vi "Dashboard Main.vi"() -> ()   [LabVIEW 2015]
uses:
  <vilib>/Utility/miscctls.llb/LVRowAndColumnTypeDef.ctl
  <vilib>/event_ctls.llb/eventvkey.ctl
  <vilib>/Rock Robotics/Network Tables/NT Read Boolean.vi
  <vilib>/Rock Robotics/WPI/Dashboard/WPI_DashboardLogging Global.vi
  <vilib>/Utility/config.llb/Write Key (String).vi
  <vilib>/Utility/config.llb/Write Key (I32).vi
  <vilib>/Utility/config.llb/NI_LVConfig.lvlib
panel:
  out "Camera Image":T1(plugin-control)
  in  "Background":bool
  in  "TCP":refnum<k5>
  in  "Vision":u16(ring) items=["Camera Off", "USB Camera SW", "USB Camera HW", "IP Camera"]
  out "Camera IP":string
  out "Image Message":string="Timeout in Camera Communications"
  in  "Dashboard Tab":T2(tab)
  in  "AUTO Start Delay":dbl
  in  "AUTO Modes":T3(radio)
  in  "Select Auto":string(combo)
  out "NT Connection":bool
  in  "Camera Settings":T4={"Frame Rate"=30, "Compression"=30, "Size"=1} {"Frame Rate" scale=1.0..30.0; "Size" items=["640x480", "320x240", "160x120"]}
  out "Mode":T5(ring)=enum."Auto Disabled"
  in  "DB Camera Config":bool
  out "fps":dbl format="%#.1g"
  out "Mbps":dbl format="%#.1g"
  out "Mbps LED":bool
  in  "Rec Mode":enum32{"Stop", "Record", "Playback"}(radio)
  in  "DB/String 9":string
  in  "DB/String 8":string
  in  "DB/String 7":string
  in  "DB/String 6":string
  in  "DB/String 5":string
  in  "DB/String 4":string
  in  "DB/String 3":string
  in  "DB/String 2":string
  in  "DB/String 1":string
  in  "DB/String 0":string
  in  "DB/Slider 0":dbl(slide) scale=0.0..5.0
  in  "DB/Slider 1":dbl(slide) scale=0.0..5.0
  in  "DB/Slider 2":dbl(slide) scale=0.0..5.0
  in  "DB/Slider 3":dbl(slide) scale=0.0..5.0
  out "DB/LED 3":bool
  out "DB/LED 2":bool
  out "DB/LED 1":bool
  out "DB/LED 0":bool
  in  "DB/Button 3":bool
  in  "DB/Button 2":bool
  in  "DB/Button 1":bool
  in  "DB/Button 0":bool caption="New Name"
  out "Shooter Velocity":dbl
  in  "Shoot Duration":dbl=1000.0
  in  "Shoot speed":dbl=0.3
  out "Refreshed":bool
  in  "Refresh":bool
  out "Saved Level 3":dbl
  out "Saved Level 2":dbl
  out "Saved Level 1":dbl
  in  "Left Shooter RPM":dbl=5000.0
  out "Pot":dbl
  in  "Test Slider":dbl(slide) scale=0.0..100.0 scale format="%#_3g"
  in  "On/Off":bool caption="Solenoid"
  in  "Test Name":u16(ring) items=["Select the test to run..."]
  in  "Test Tree":string(tree)
  in  "Motor":cluster{"Value":dbl, "Enable":bool} {"Value" scale=-1.0..1.0 scale format="%#_3g"}
  out "Progress":T6 {"Test Progress" scale=0.0..100.0}
  in  "Rev/Fwd":cluster{"Forward":bool, "Reverse":bool}
  in  "Test Ring":u16(ring) items=["Monochrome", "Color"]
  out "Cmd Status":string
  in  "Execute Command":bool
  in  "Command Params":string[][](table)
  in  "Command Selection":i32(listbox)
  in  "CheckList":i32(listbox)
  out "Tree":string(tree)
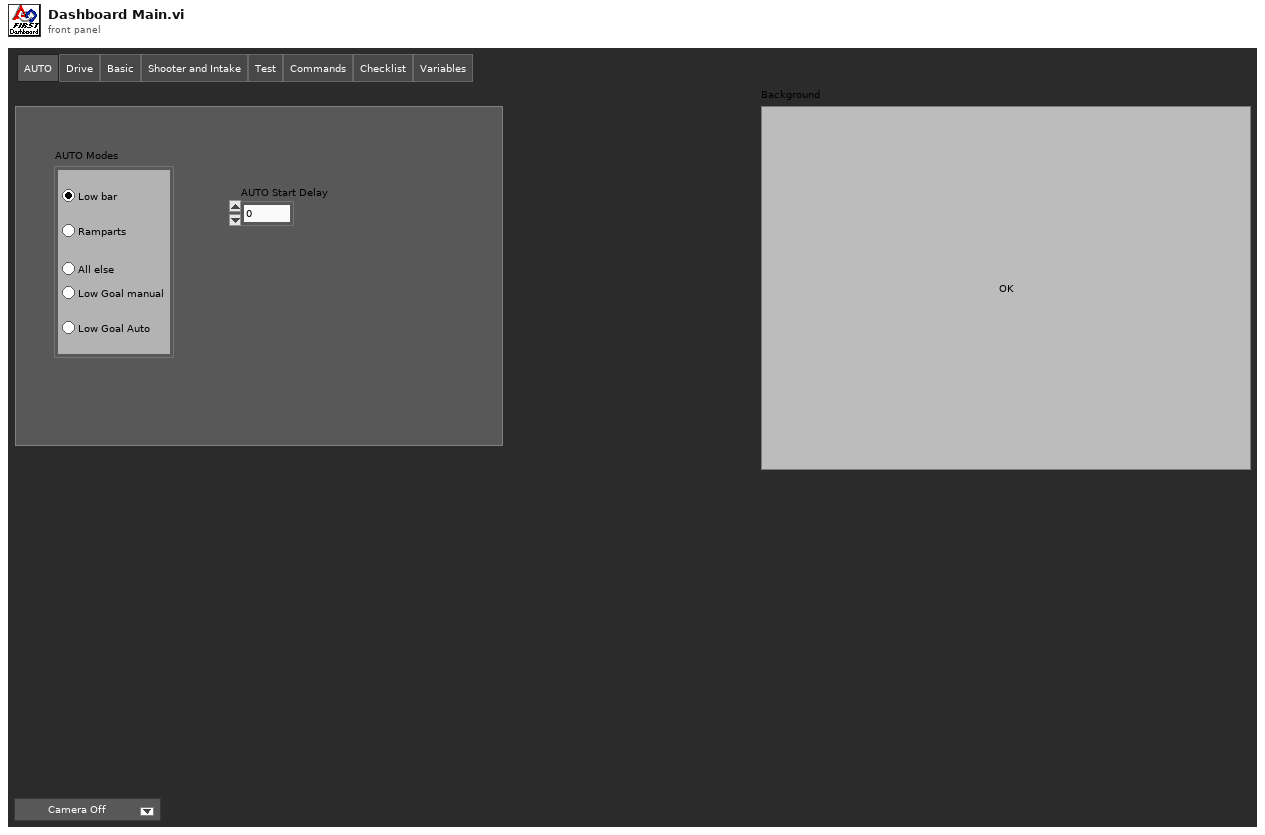
[diagram p1: front panel]
types:
  T1 = typedef "IMAQ Image.ctl" = refnum<image>
  T2 = enum32{"AUTO", "Drive", "Basic", "Shooter and Intake", "Test", "Commands", "Checklist", "Variables"}
  T3 = enum32{"Low bar", "Ramparts", "All else", "All else 2", "All else 3"}
  T4 = cluster{"Frame Rate":i32, "Compression":i32, "Size":u16}
  T5 = enum8{"Tele-Op Disabled", "Tele-Op Enabled", "Auto Disabled", "Auto Enabled", "Test Disabled", "Test Enabled", "Disconnected", "No Code", "E-Stop"}
  T6 = cluster{"Test Progress":u8, "Test Progress Text":string}
  T7 = cluster{"IDs":cluster{"RPC field ID":u16, "Unique ID":u16}, "String":string}
  T8 = enum32{"Drive", "Basic", "Custom", "Test", "Checklist", "Variables"}
  T9 = typedef "Image Type" = u32
  T10 = enum16{"open", "replace", "create", "open or create", "replace or create", "replace or create with confirmation"}
  T11 = cluster{"Camera Image":refnum<vi>, "Dashboard Tab":refnum<vi>, "Background":refnum<vi>, "Vision":refnum<vi>, "Rec Mode":refnum<vi>, "Test Slider":refnum<vi>, "On/Off ":refnum<vi>, "Test Ring":refnum<vi>, "Rev/Fwd":refnum<vi>, "Test Name":refnum<vi>, "Motor":refnum<vi>, "Progress":refnum<vi>, "CheckList":refnum<vi>, "Tree":refnum<vi>, "Test Tree":refnum<vi>, "Command Params":refnum<vi>, "Command Selection":refnum<vi>, "Execute Command":refnum<vi>, "Cmd Status":refnum<vi>}
  T12 = typedef "NI_LVConfig.lvlib/Config Data RefNum.ctl" = refnum<k1>
  T13 = cluster{"Error Strings":string, "Disable Counts":cluster{u16, u16}, "Rail Faults":cluster{u16, u16, u16}, "Robot IP":string, "DB Mode":u8, "Event Info":cluster{"Name":string, "Type":u8, "Number":u16, "Replay":u8}, "Camera Addr":string}
  T14 = cluster{"Storage":cluster{"Disk Free":u64, "RAM Block":u32, "RAM free":u32}, "CPU Utilization":cluster{"CPU % ISR":sgl, "CPU % Time Crit":sgl, "CPU % Timed Str":sgl, "CPU % High":sgl, "CPU % Above":sgl, "CPU % Normal":sgl, "CPU % Low":sgl}, "CAN":cluster{"% Bus Utilization":sgl, "Bus Off Cnt":u32, "TX_FIFO Full Cnt":u32, "Receive Error Cnt":u8, "Transmit Error Cnt":u8}, "HID":cluster{"HID Outputs":u32, "Rumble Low":u16, "Rumble High":u16}[]}
  T15 = cluster{"Status bits":cluster{"Test Mode":bool, "Autonomous":bool, "Enabled":bool, "Code Start":bool, "Brownout":bool, "Reserved 2":bool, "Reserved 3":bool, "E-Stop":bool}, "Code Trace":cluster{"Disabled":bool, "TeleOp":bool, "Auto":bool, "Test":bool}, "Controller Type":enum16{"unknown", "cRIO", "roboRio"}, "Code?":enum16{"unknown", "noCode", "code"}, "Battery V":dbl}
  T16 = cluster{"Control Bits":cluster{"TestMode":bool, "Autonomous":bool, "Enabled":bool, "FMS Present":bool, bool, bool, bool, "E-Stop":bool}, "Team Station ":u8, "Countdown":sgl, "Joystick Values":cluster{"Axes":dbl[], "Buttons":bool[], "POVs":i16[]}[]}
  T17 = cluster{"Operation":enum16{"Update", "Clear"}, "Color Box":u32}[]
  T18 = typedef "eventvkey.ctl" = enum16{"ASCII", "Enter", "Return", "Shift", "Ctrl", "Alt", "Cmd", "Opt", "Caps", "NumLock", "Clear", "Break", "Up", "Down", "Left", "Right", "Insert", "Delete", "Home", "End", "PageUp", "PageDown", "Escape", "Help", "Pause", "ScrollLock", "F1", "F2", "F3", "F4", "F5", "F6", "F7", "F8", "F9", "F10", "F11", "F12", "F13", "F14", "F15", "F16", "F17", "F18", "F19", "F20", "F21", "F22", "F23", "F24", "Play", "VolumeUp", "VolumeDown", "Mute", "Two Byte Char"}
  T19 = cluster{"Image Size":bool, "Image Type":bool, "Pixel Value":bool, "ROI Information":bool, "Zoom Factor":bool}
  T20 = enum8{"Enabled", "Disabled", "Disabled and Grayed Out"}
  T21 = cluster{"Operation":enum16{"Update", "Clear"}, "Color Box":u32}
  T22 = typedef "LVRowAndColumnTypeDef.ctl" = cluster{"Row":i32, "Column":i32}
  T23 = cluster{"Shift":bool, "Ctrl":bool, "Alt":bool, "Cmd":bool, "Opt":bool}
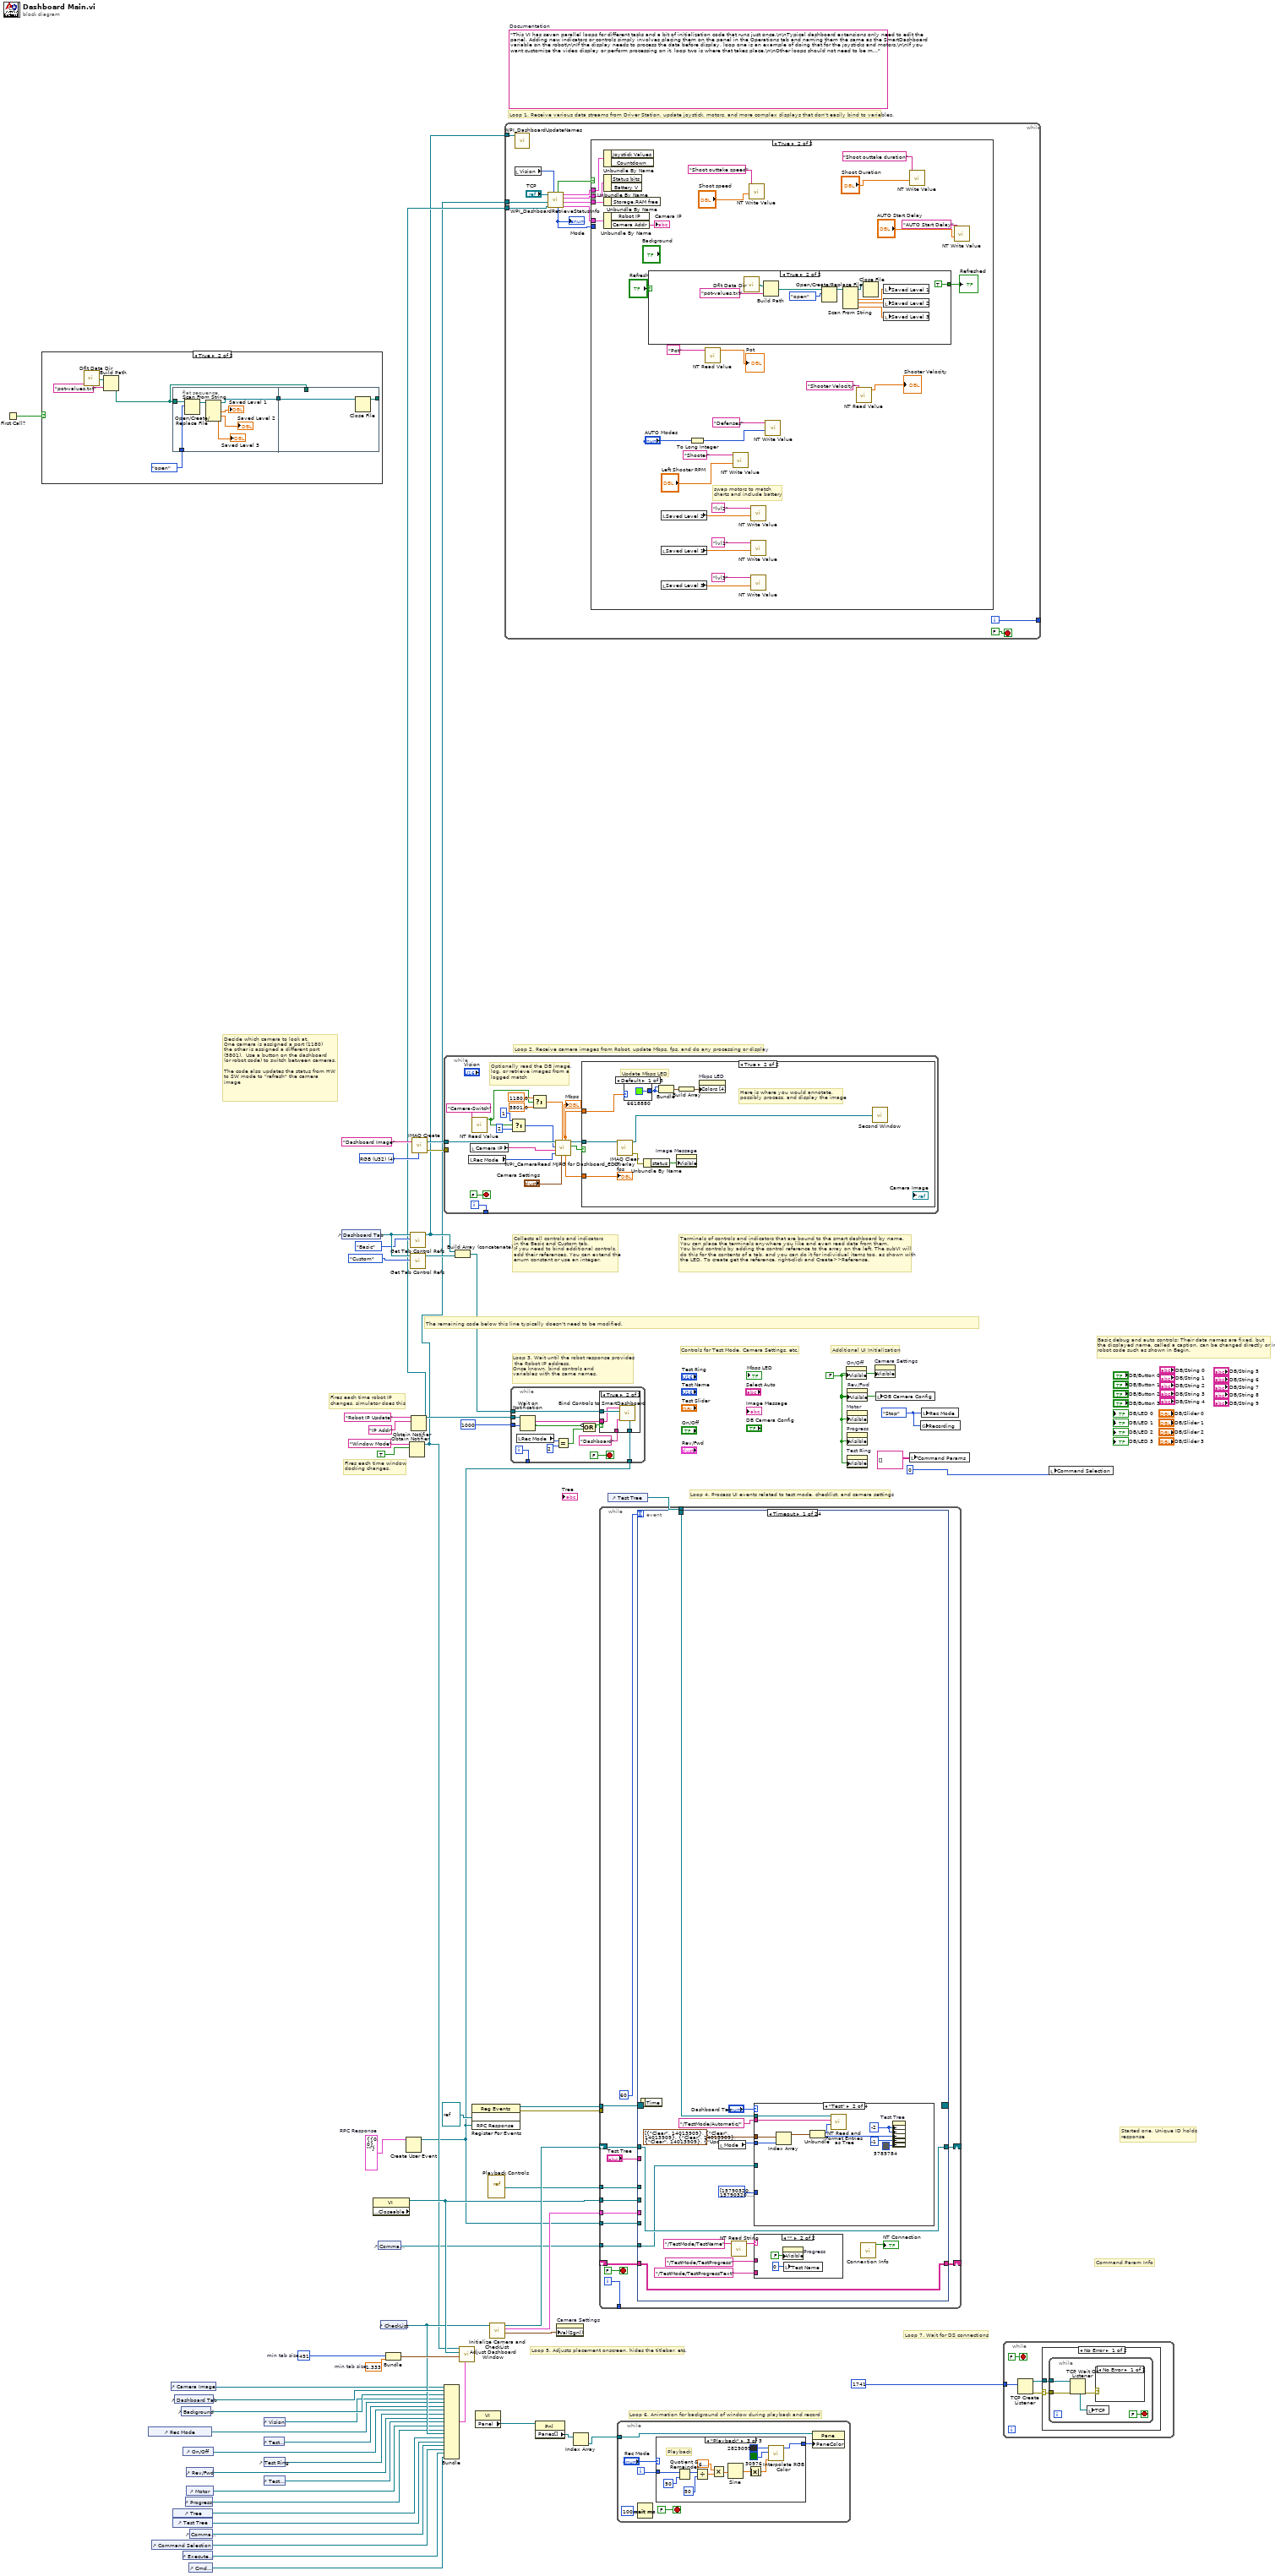
[diagram p0: block diagram]
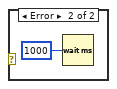
[diagram p3: hidden frame]
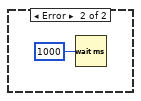
[diagram p4: hidden frame]
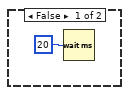
[diagram p5: hidden frame]
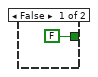
[diagram p6: hidden frame]
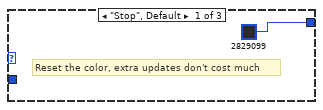
[diagram p7: hidden frame]
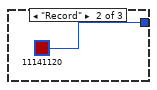
[diagram p8: hidden frame]
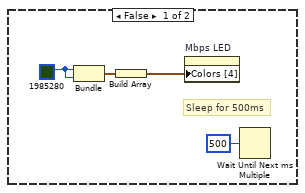
[diagram p10: hidden frame]
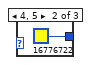
[diagram p11: hidden frame]
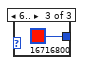
[diagram p12: hidden frame]
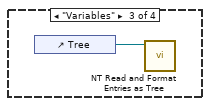
[diagram p14: hidden frame]
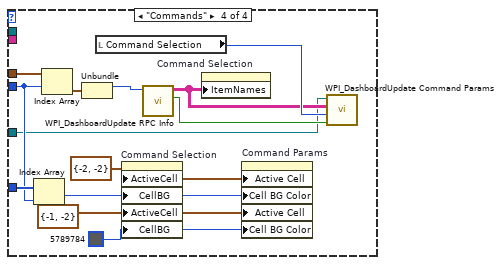
[diagram p15: hidden frame]
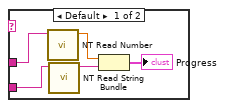
[diagram p16: hidden frame]
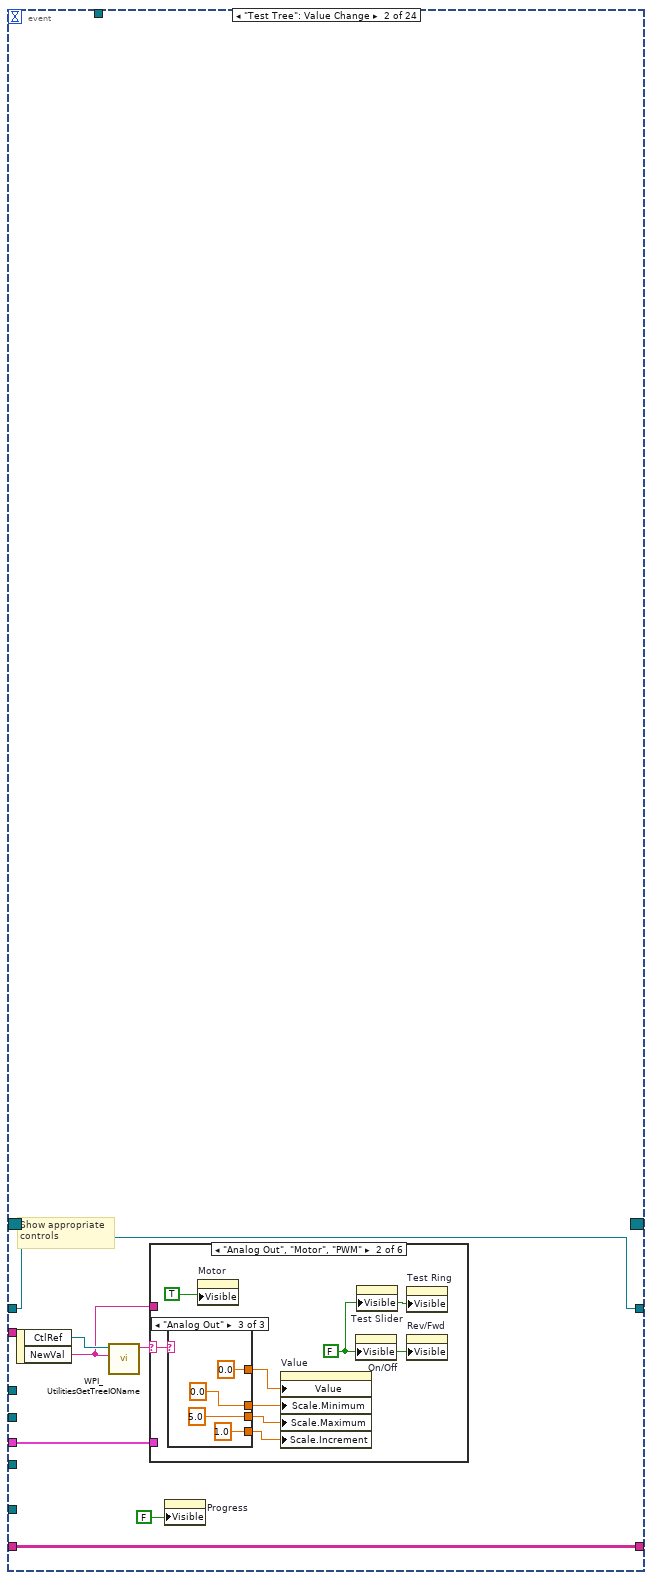
[diagram p17: hidden frame]
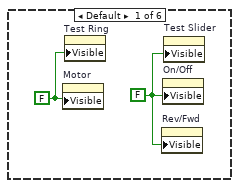
[diagram p18: hidden frame]
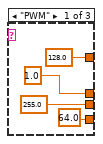
[diagram p19: hidden frame]
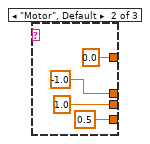
[diagram p20: hidden frame]
diagram:
  w12 = T7 {"IDs"={"RPC field ID"=0, "Unique ID"=0}, "String"=""}  # RPC Response
  w35 = 491  # min tab size
  w34 = 1.333  # min tab size
  w41 = enum32{"Stop", "Record", "Playback"}."Stop" ("Rec Mode")
  w19 = FALSE ("Visible")
  (unwired) "This VI has seven parallel loops for different tasks and a bit of initialization code that runs just once.\n\nTypical dashboard extensions only need to edit the panel. Adding new indicators or controls simply involves placing them on the panel in the Operations tab and naming them the same as the SmartDashboard variable on the robot\n\nIf the display needs to process the data before display, loop one is an example of doing that for the joysticks and motors.\n\nIf you want customize the video display or perform processing on it, loop two is where that takes place.\n\nOther loops should not need to be modified. They are pretty standard, and document the task they perform."  # Documentation
  w61 = T9 4 items=["Grayscale (U8)", "Grayscale (I16)", "Grayscale (SGL)", "Complex (CSG)", "RGB (U32)", "HSL (U32)", "RGB (U64)"] ("Image Type")
  # "Decide which camera to look at.\nOne camera is assigned a port (1180)\nthe other is assigned a different port\n(5801).  Use a button on the dashboard\n(or robot code) to switch between cameras.\n\nThe code also updates the status from HW\nto SW mode to \"refresh\" the camera\nimage"
  # "Command Param Info"
  # "Started one, Unique ID holds\nresponse"
  # "Loop 7. Wait for DS connections"
  # "Basic debug and auto controls: Their data names are fixed, but\nthe displayed name, called a caption, can be changed directly or in\nrobot code such as shown in Begin."
  # "Controls for Test Mode, Camera Settings, etc."
  # "Additional UI Initialization"
  # "Loop 6. Animation for background of window during playback and record"
  # "Fires each time robot IP\nchanges, simulator does this"
  # "Fires each time window\ndocking changes."
  # "Collects all controls and indicators\nin the Basic and Custom tab.\nIf you need to bind additional controls,\nadd their references. You can extend the\nenum constant or use an integer."
  # "The remaining code below this line typically doesn't need to be modified."
  # "Loop 4. Process UI events related to test mode, checklist, and camera settings"
  # "Terminals of controls and indicators that are bound to the smart dashboard by name.\nYou can place the terminals anywhere you like and even read data from them.\nYou bind controls by adding the control reference to the array on the left. The subVI will\ndo this for the contents of a tab, and you can do it for individual items too, as shown with\nthe LED. To create get the reference, right-click and Create>>Reference."
  # "Loop 3. Wait until the robot response provides\n the Robot IP address.\nOnce known, bind controls and\nvariables with the same names."
  # "Loop 5. Adjusts placement onscreen, hides the titlebar, etc."
  # "Loop 1. Receive various data streams from Driver Station, update joystick, motors, and more complex displays that don't easily bind to variables."
  # "Loop 2. Receive camera images from Robot, update Mbps, fps, and do any processing or display"
  n1 = First Call?() -> (First Call?: T/F=w1:bool)
  n2 = case shown="True" w1 {
    frame False {
    }
    frame True {
      n3 = call <vilib>:"Dflt Data Dir.vi"() -> ("App:Default Data Directory"=w66:path)
      n4 = Build Path(base path=w66, name or relative path="pot-values.txt") -> (appended path=w63:path)
      n5 = flat-sequence {
        tunnel: w63 -> [w73]
        tunnel: T10."open" ("operation (0:open)") -> [w72]
        tunnel: [w67] -> w62
        tunnel: [w75] -> _
        tunnel: w63 -> [_]
        tunnel: w62 -> [w74]
        frame #0 {
          n6 = Open/Create/Replace File(file path (use dialog)=w73, operation (0:open)=w72) -> (refnum out=w71:refnum<file>)  [unwired: 4 in, 2 out]
          n7 = Scan From String(w71) -> (w67:refnum<file>, output 1=→"Saved Level 1":dbl, output 2=→"Saved Level 2":dbl, output 3=→"Saved Level 3":dbl)  [unwired: 5 in, 1 out]
        }
        frame #1 {
          n8 = Close File(refnum=w74) -> (path=w75:path)  [unwired: 1 in, 1 out]
        }
      }
    }
  }
  n9 = control-ref of="Rec Mode"() -> (w25:refnum<vi>)
  n10 = control-ref of="Command Selection"() -> (w11:refnum<vi>)
  n11 = control-ref of="Camera Image"() -> (w3:refnum<vi>)
  n12 = control-ref of="Tree"() -> (w29:refnum<vi>)
  n13 = control-ref of="Test Tree"() -> (w28:refnum<vi>)
  n14 = control-ref of="Dashboard Tab"() -> (w36:refnum<vi>)
  n15 = control-ref of="Background"() -> (w5:refnum<vi>)
  n16 = control-ref of="Execute Command"() -> (w13:refnum<vi>)
  n17 = control-ref of="On/Off"() -> (w23:refnum<vi>)
  n18 = control-ref of="Progress"() -> (w20:refnum<vi>)
  n19 = control-ref of="Rev/Fwd"() -> (w21:refnum<vi>)
  n20 = control-ref of="Motor"() -> (w26:refnum<vi>)
  n21 = control-ref of="Cmd Status"() -> (w7:refnum<vi>)
  n22 = control-ref of="Command Params"() -> (w14:refnum<vi>)
  n23 = control-ref of="Test Slider"() -> (w24:refnum<vi>)
  n24 = control-ref of="Vision"() -> (w4:refnum<vi>)
  n25 = control-ref of="Test Ring"() -> (w22:refnum<vi>)
  n26 = control-ref of="Test Name"() -> (w27:refnum<vi>)
  n27 = control-ref of="Dashboard Tab"() -> (w39:refnum<vi>)
  n28 = property class="VI" props=["Front Panel.Closeable"]() -> (reference out=w40:refnum<vi>)  [unwired: 2 in, 2 out]
  n29 = control-ref of="Command Params"() -> (w6:refnum<vi>)
  n30 = control-ref of="CheckList"() -> (w30:refnum<vi>)
  n31 = Bundle("min tab size"=w35, "min tab size"=w34) -> (w33:cluster{"min tab size":i32, "min tab size":dbl})  [unwired: 1 in]
  n32 = Create User Event(user event datatype=w12) -> (user event=w8:refnum<user-event>)  [unwired: 1 in, 1 out]
  n33 = Obtain Notifier(name (unnamed)="Window Mode", notification data type=TRUE) -> (notifier out=w16:refnum<notifier>)  [unwired: 2 in, 2 out]
  n34 = call <vilib>:"Get Tab Control Refs.vi"("Page Index"=T8."Basic" ("Dashboard Tab"), "TabControl in"=w39) -> ("ControlsOnPage"=w17:refnum<vi>[])  [unwired: 9 in]
  n35 = call <vilib>:"Get Tab Control Refs.vi"("Page Index"=T8."Custom" ("Dashboard Tab"), "TabControl in"=w39) -> ("ControlsOnPage"=w38:refnum<vi>[])  [unwired: 9 in]
  n36 = Obtain Notifier(name (unnamed)="Robot IP Update", notification data type="IP Addr" ("name (unnamed)")) -> (notifier out=w18:refnum<notifier>)  [unwired: 2 in, 2 out]
  n37 = call "IMAQ Create"("Image Name"="Dashboard Image", "Image Type"=w61) -> ("New Image"=w59:T1, "error out"=w58:errorcluster)  [unwired: 2 in, 1 out]
  n38 = while {
    tunnel: w59 -> [w91]
    tunnel: w58 -> [_]
    tunnel: [w92] -> _
    i -> [w92]
    stop <- FALSE stop-if-true
    # "Optionally read the DB image,\nlog, or retrieve images from a\nlogged match"
    n39 = local read "Rec Mode"() -> (w86:enum32{"Stop", "Record", "Playback"})
    n40 = local read "Camera IP"() -> (w85:string)
    n41 = call-poly <vilib>:"NT Read Value.vi"("Name"="Camera-Switch") -> ("Boolean"=w76:bool)  [unwired: 9 in, 1 out]
    n42 = Select(t=1, s=w76, f=2) -> (s? t:f=w81:i32)
    n43 = Select(t=1180.0, s=w76, f=5801.0) -> (s? t:f=w80:dbl)
    n44 = call "WPI_CameraRead MJPG for Dashboard_EDIT.vi"("Camera Settings"="Camera Settings", "Camera Port"=w80, "Rec Mode"=w86, "Camera IP"=w85, "Camera Mode"=w81, "Refnum in"=w91) -> ("Active"=w89:bool, "Refnum out"=w90:T1, "FPS"=w88:dbl, "Bandwidth (Mbps)"=w84:dbl)  [unwired: 2 in]
    "Mbps" <- w84
    n45 = case shown="True" w89 {
      tunnel: w90 -> [_ w101]
      tunnel: w84 -> [_ w100]
      tunnel: w88 -> [_ w99]
      frame False {
        w94 = u32 1985280 ("Color Box")
        # "Sleep for 500ms"
        n46 = Bundle("Color Box"=w94, "Color Box"=w94) -> (w96:cluster{"Color Box":u32, "Color Box":u32})  [unwired: 1 out]
        n47 = Build Array(w96) -> (w95:cluster{"Color Box":u32, "Color Box":u32}[])
        n48 = property on="Mbps LED" class="Bool (strict)"("Colors [4]"=w95) -> ()  [unwired: 2 in, 2 out]
        n49 = Wait Until Next ms Multiple(millisecond multiple=u32 500) -> ()  [unwired: 1 out]
      }
      frame True {
        # "Here is where you would annotate,\npossibly process, and display the image"
        # "Update Mbps LED"
        n50 = call "IMAQ Clear Overlay"("Image"=w101) -> ("error out"=w105:errorcluster, "Image Out"=w98:T1)  [unwired: 2 in, 7 out]
        n51 = case shown="Default" w100 {
          tunnel: [u32 6618880 ("Color Box") u32 16776722 ("Color Box") u32 16716800 ("Color Box")] -> w102
          frame Default {
          }
          frame 4, 5 {
          }
          frame 6.. {
          }
        }
        n52 = Unbundle By Name(w105) -> ("status"=w106:bool)
        n53 = Bundle("Color Box"=w102, "Color Box"=w102) -> (w104:cluster{"Color Box":u32, "Color Box":u32})  [unwired: 1 out]
        n54 = property on="Image Message" class="Str"("Visible"=w106) -> ()  [unwired: 2 in, 2 out]
        n55 = Build Array(w104) -> (w103:cluster{"Color Box":u32, "Color Box":u32}[])
        n56 = property on="Mbps LED" class="Bool (strict)"("Colors [4]"=w103) -> ()  [unwired: 2 in, 2 out]
        n57 = call "Second Window.vi"("Input Camera Image"=w98) -> ()  [unwired: 1 in]
        "fps" <- w99
      }
    }
  }
  n58 = Bundle("Camera Image"=w3, "Dashboard Tab"=w36, "Background"=w5, "Vision"=w4, "Rec Mode"=w25, "Test Slider"=w24, "On/Off"=w23, "Test Ring"=w22, "Rev/Fwd"=w21, "Test Name"=w27, "Motor"=w26, "Progress"=w20, "CheckList"=w30, "Tree"=w29, "Test Tree"=w28, "Command Params"=w14, "Command Selection"=w11, "Execute Command"=w13, "Cmd Status"=w7) -> (w2:T11)  [unwired: 1 in]
  n59 = Build Array (concatenate)(w17, w38) -> (w37:refnum<vi>[])
  n60 = call "Adjust Dashboard Window.vi"("Sizing Refnums"=w2, "Size Constraints"=w33, "VI"=w40, "WIn Mode"=w16) -> ()  [unwired: 8 in]
  n61 = register-events(refnum<vi> refnum, w8) -> (reference out=w45:refnum<event-registration>, error out=w44:errorcluster)  [unwired: 2 in]
  n62 = property class="VI"() -> ("Panel"=w48:refnum<vi>)  [unwired: 2 in, 2 out]
  n63 = vi-ref "Playback Controls.vi"() -> (w46:refnum<vi>)
  n64 = call "Initialize Camera and CheckList.vi"("ListBox in"=w30) -> ("Cluster"=w52:cluster{"value":i32, "value":i32, "index":i32}, "Array"=w53:cluster{string[]}[], "File Refnum"=w51:T12)  [unwired: 8 in]
  n65 = while {
    tunnel: [w121] -> _
    tunnel: w18 -> [w115]
    tunnel: w17 -> [w114]
    tunnel: w16 -> [w110]
    i -> [w121]
    stop <- FALSE stop-if-true
    n66 = call <vilib>:"WPI_DashboardUpdateNames.vi"("Controls on Tab"=w114) -> ()  [unwired: 11 in]
    n67 = local read "Vision"() -> (w112:u16)
    n68 = call <vilib>:"WPI_DashboardRetrieveStatusInfo.vi"("Vision"=w112, "Binding Refnum"=w115, "Window Mode Notifier"=w110, "TCP Cnx"="TCP") -> ("Power and Errors"=w116:T13, "Robot Metrics"=w119:T14, "Status Info"=w120:T15, "Control Info"=w117:T16, "Robot Mode"=w113:T5, "Process?"=w118:bool)  [unwired: 2 in]
    "Mode" <- w113
    n69 = case shown="True" w118 {
      tunnel: w120 -> [_ w151]
      tunnel: w119 -> [_ w150]
      tunnel: w117 -> [_ w149]
      tunnel: w116 -> [_ w148]
      tunnel: w113 -> [_ _]
      frame False {
        n70 = Wait (ms)(milliseconds to wait=u32 20) -> ()  [unwired: 1 out]
      }
      frame True {
        # "swap motors to match\ncharts and include battery"
        n71 = Unbundle By Name(w149) -> ()  [unwired: 2 out]
        n72 = Unbundle By Name(w151) -> ()  [unwired: 2 out]
        n73 = Unbundle By Name(w150) -> ()  [unwired: 1 out]
        n74 = Unbundle By Name(w148) -> ("Camera Addr"=→"Camera IP":string)  [unwired: 1 out]
        n75 = case shown="True" "Refresh" {
          tunnel: [FALSE TRUE] -> w133
          frame False {
          }
          frame True {
            n76 = call <vilib>:"Dflt Data Dir.vi"() -> ("App:Default Data Directory"=w161:path)
            n77 = Build Path(base path=w161, name or relative path="pot-values.txt") -> (appended path=w159:path)
            n78 = Open/Create/Replace File(file path (use dialog)=w159, operation (0:open)=T10."open") -> (refnum out=w162:refnum<file>)  [unwired: 4 in, 2 out]
            n79 = Scan From String(w162) -> (w154:refnum<file>, output 1=w155:dbl, output 2=w157:dbl, output 3=w156:dbl)  [unwired: 5 in, 1 out]
            n80 = Close File(refnum=w154) -> ()  [unwired: 1 in, 2 out]
            n81 = local write "Saved Level 1"(w155) -> ()
            n82 = local write "Saved Level 2"(w157) -> ()
            n83 = local write "Saved Level 3"(w156) -> ()
          }
        }
        "Refreshed" <- w133
        n84 = local read "Saved Level 2"() -> (w135:dbl)
        n85 = local read "Saved Level 1"() -> (w134:dbl)
        n86 = local read "Saved Level 3"() -> (w136:dbl)
        n87 = To Long Integer(number="AUTO Modes") -> (32bit integer=w138:i32)
        n88 = call-poly <vilib>:"NT Read Value.vi"("Name"="Pot") -> ("Numeric"=→"Pot":dbl)  [unwired: 9 in, 1 out]
        n89 = call-poly <vilib>:"NT Write Value.vi"("Numeric"="Left Shooter RPM", "Name"="Shooter") -> ()  [unwired: 9 in, 1 out]
        n90 = call-poly <vilib>:"NT Write Value.vi"("Numeric"="Shoot speed", "Name"="Shoot outtake speed") -> ()  [unwired: 9 in, 1 out]
        n91 = call-poly <vilib>:"NT Write Value.vi"("Numeric"=w135, "Name"="lvl2") -> ()  [unwired: 9 in, 1 out]
        n92 = call-poly <vilib>:"NT Write Value.vi"("Numeric"=w134, "Name"="lvl1") -> ()  [unwired: 9 in, 1 out]
        n93 = call-poly <vilib>:"NT Write Value.vi"("Numeric"=w136, "Name"="lvl3") -> ()  [unwired: 9 in, 1 out]
        n94 = call-poly <vilib>:"NT Write Value.vi"("Numeric"=w138, "Name"="Defenses") -> ()  [unwired: 9 in, 1 out]
        n95 = call-poly <vilib>:"NT Read Value.vi"("Name"="Shooter Velocity") -> ("Numeric"=→"Shooter Velocity":dbl)  [unwired: 9 in, 1 out]
        n96 = call-poly <vilib>:"NT Write Value.vi"("Numeric"="Shoot Duration", "Name"="Shoot outtake duration") -> ()  [unwired: 9 in, 1 out]
        n97 = call-poly <vilib>:"NT Write Value.vi"("Numeric"="AUTO Start Delay", "Name"="AUTO Start Delay") -> ()  [unwired: 9 in, 1 out]
      }
    }
  }
  n98 = while {
    tunnel: w37 -> [w175]
    tunnel: w18 -> [w173]
    tunnel: [w171] -> _
    tunnel: u32 1000 ("milliseconds to wait") -> [w170]
    tunnel: w8 -> [w163]
    i -> [w171]
    stop <- FALSE stop-if-true
    n99 = local read "Rec Mode"() -> (w166:enum32{"Stop", "Record", "Playback"})
    n100 = Wait on Notification(notifier=w173, timeout in ms (-1)=w170) -> (notification=w172:string, timed out?=w168:bool)  [unwired: 2 in, 2 out]
    n101 = Equal?(x=w166, y=u16 2 ("Rec Mode")) -> (x = y?=w167:bool)
    n102 = Compound Arithmetic op=OR(invert w168, w167) -> (w169:bool)
    n103 = case shown="True" w169 {
      tunnel: w175 -> [_ w179]
      tunnel: w172 -> [_ w178]
      tunnel: "Dashboard" -> [_ w177]
      tunnel: w163 -> [_ w176]
      frame False {
      }
      frame True {
        n104 = call <vilib>:"Bind Controls to SmartDashboard.vi"("RPC ref"=w176, "Client Name"=w177, "Bound Control Refs"=w179, "Server IP Address"=w178) -> ()  [unwired: 8 in]
      }
    }
  }
  n105 = property class="Pnl"(reference=w48) -> ("Panes[]"=w49:refnum<vi>[])  [unwired: 1 in, 2 out]
  n106 = property on="Camera Settings" class="Clust (strict)"("Val(Sgnl)"=w52) -> ()  [unwired: 2 in, 2 out]
  n107 = Index Array(array=w49) -> (element=w47:refnum<vi>)  [unwired: 1 in]
  n108 = control-ref of="Test Tree"() -> (w50:refnum<vi>)
  n109 = while {
    tunnel: w53 -> [w191]
    shift-right: [w190] -> _
    shift-left: w51 -> [w189]
    tunnel: [w188] -> _
    tunnel: w50 -> [w187]
    tunnel: w46 -> [w186]
    tunnel: w45 -> [w185]
    tunnel: w44 -> [_]
    tunnel: w40 -> [w184]
    tunnel: w8 -> [w183]
    tunnel: w6 -> [w182]
    shift-right: [w181] -> _
    shift-left: _ -> [w180]
    i -> [w188]
    stop <- FALSE stop-if-true
    n110 = event shown="[0] Timeout" {
      selector: w185 -> [_ _ _ _ _ _ _ _ _ _ _ _ _ _ _ _ _ _ _ _ _ _ _ _]
      dyn-events: [_ _ _ _ _ _ _ _ _ _ _ _ _ _ _ _ _ _ w498 _ _ _ _ _] -> _
      timeout: u32 60 ("milliseconds to wait") -> [_ _ _ _ _ _ _ _ _ _ _ _ _ _ _ _ _ _ _ _ _ _ _ _]
      tunnel: w187 -> [w204 _ _ _ _ _ _ _ _ _ _ _ _ _ _ _ _ _ _ _ _ _ _ _]
      tunnel: "Test Tree" -> [_ _ _ _ _ _ _ _ _ _ _ _ _ w463 w472 w475 w480 w489 _ _ _ _ _ _]
      tunnel: w191 -> [_ w242 _ _ _ _ _ _ _ _ _ w425 w456 _ _ _ _ _ _ _ _ _ _ _]
      tunnel: [w201 w241 w345 w351 w361 w365 w371 w383 w391 w397 w410 w424 w449 w462 w470 w474 w479 w488 w500 w516 w518 w526 w537 w542] -> w190
      tunnel: w189 -> [w201 w241 w345 w351 w361 w365 w371 w383 w391 w397 w410 w423 w449 w462 w470 w474 w479 w488 w500 w516 w518 w526 w537 w542]
      tunnel: w186 -> [_ _ _ _ _ _ _ _ _ _ _ _ _ _ _ _ _ _ w501 _ w521 _ _ _]
      tunnel: w184 -> [_ _ _ _ _ _ _ _ _ _ _ _ _ _ _ _ _ _ w496 _ _ _ _ _]
      tunnel: w183 -> [_ _ _ _ _ _ _ _ _ _ _ _ _ _ _ _ _ _ w494 _ _ _ _ _]
      tunnel: w182 -> [w196 _ _ _ _ _ w369 _ _ _ _ _ _ _ _ _ _ _ _ _ _ _ _ _]
      tunnel: [w195 w240 w344 w350 w360 w366 w367 w377 w388 w396 w409 w422 w448 w461 w469 w473 w478 w487 w493 w514 w517 w522 w530 w543] -> w181
      tunnel: w180 -> [w195 w240 w344 w350 w360 w366 w367 _ _ w396 w409 w422 w448 w461 w469 w473 w478 w487 w493 w514 w517 w522 w530 w543]
      event Timeout {
        n111 = event-data() -> ()  [unwired: 1 in, 1 out]
        n112 = local read "Mode"() -> (w198:T5)
        n113 = call <vilib>:"NT Read String.vi"("Name"="/TestMode/TestName") -> ("String"=w207:string)  [unwired: 9 in, 1 out]
        n114 = case shown="\"Test\"" "Dashboard Tab" {
          tunnel: w204 -> [_ w218 _ _]
          tunnel: "/TestMode/Automatic/" ("Name Pattern") -> [_ w217 _ _]
          tunnel: T17 [{"Operation"=enum."Clear", "Color Box"=14013909}, {"Operation"=enum."Clear", "Color Box"=14013909}, {"Operation"=enum."Clear", "Color Box"=14013909}, {"Operation"=enum."Clear", "Color Box"=14013909}, {"Operation"=enum."Update", "Color Box"=14013909}, {"Operation"=enum."Update", "Color Box"=16777215}, {"Operation"=enum."Clear", "Color Box"=14013909}, {"Operation"=enum."Clear", "Color Box"=14013909}, {"Operation"=enum."Clear", "Color Box"=14013909}] -> [_ w210 _ w227]
          tunnel: w198 -> [_ w209 _ w226]
          tunnel: u32[] [15790320, 15790320, 15790320, 15790320, 16777215, 16777215, 15790320, 15790320, 15790320] -> [_ _ _ w232]
          tunnel: w196 -> [_ _ _ w220]
          frame "Shooter and Intake", Default {
          }
          frame "Test" {
            w216 = -2 ("Active Item:Row Number")
            n115 = Index Array(array=w210, index=w209) -> (element=w211:T21)
            n116 = Unbundle(w211) -> ("Operation"=w212:enum16{"Update", "Clear"}, "Color Box"=w213:u32)
            n117 = call <vilib>:"NT Read and Format Entries as Tree.vi"("Operation"=w212, "Name Pattern"=w217, "Tree Refnum"=w218) -> ()  [unwired: 7 in, 2 out]
            n118 = property on="Test Tree" class="Tree (strict)"("Active Item Row Number"=w216, "ActiveColNum"=w216, "CellBG"=w213, "Active Item Row Number"=-1 ("Active Item:Row Number"), "CellBG"=u32 5789784 ("Color Box")) -> ()  [unwired: 2 in, 2 out]
          }
          frame "Variables" {
            n119 = control-ref of="Tree"() -> (w219:refnum<vi>)
            n120 = call <vilib>:"NT Read and Format Entries as Tree.vi"("Tree Refnum"=w219) -> ()  [unwired: 9 in, 2 out]
          }
          frame "Commands" {
            w228 = u32 5789784 ("Color Box")
            w229 = T22 {"Row"=-1, "Column"=-2} ("Active Cell:Active Cell")
            w231 = T22 {"Row"=-2, "Column"=-2} ("Active Cell:Active Cell")
            n121 = Index Array(array=w232, index=w226) -> (element=w230:u32)
            n122 = Index Array(array=w227, index=w226) -> (element=w225:T21)
            n123 = Unbundle(w225) -> ("Operation"=w224:enum16{"Update", "Clear"})  [unwired: 1 out]
            n124 = local read "Command Selection"() -> (w223:i32)
            n125 = property on="Command Selection" class="MCListbox (strict)"("ActiveCell"=w231, "CellBG"=w230, "ActiveCell"=w229, "CellBG"=w228) -> ()  [unwired: 2 in, 2 out]
            n126 = call <vilib>:"WPI_DashboardUpdate RPC Info.vi"("Operation"=w224) -> ("update"=w222:bool, "commands"=w221:string[][])  [unwired: 9 in]
            n127 = property on="Command Selection" class="MCListbox (strict)"("ItemNames"=w221) -> ()  [unwired: 2 in, 2 out]
            n128 = property on="Command Params" class="Tbl (strict)"("Active Cell"=w231, "Cell BG Color"=w230, "Active Cell"=w229, "Cell BG Color"=w228) -> ()  [unwired: 2 in, 2 out]
            n129 = call <vilib>:"WPI_DashboardUpdate Command Params.vi"("Update"=w222, "NewVal"=w223, "Commands"=w221, "Param Tbl"=w220) -> ()  [unwired: 7 in, 1 out]
          }
        }
        n130 = case shown="\"\"" w207 {
          tunnel: "/TestMode/TestProgress" ("Name") -> [w234 _]
          tunnel: "/TestMode/TestProgressText" ("Name") -> [w233 _]
          frame Default {
            n131 = call <vilib>:"NT Read Number.vi"("Name"=w234) -> ("Numeric"=w235:dbl)  [unwired: 9 in, 1 out]
            n132 = call <vilib>:"NT Read String.vi"("Name"=w233) -> ("String"=w236:string)  [unwired: 9 in, 1 out]
            n133 = Bundle("Numeric"=w235, "String"=w236) -> (→"Progress":cluster{"Numeric":dbl, "String":string})  [unwired: 1 in]
          }
          frame "" {
            n134 = property on="Progress" class="Clust (strict)"("Visible"=FALSE) -> ()  [unwired: 2 in, 2 out]
            n135 = local write "Test Name"(u16 0) -> ()
          }
        }
        n136 = call <vilib>:"Connextion Info.vi"() -> ("Connected"=→"NT Connection":bool)  [unwired: 10 in, 1 out]
      }
      event "Test Tree": Value Change {
        # "Show appropriate\ncontrols"
        n137 = event-data() -> ("CtlRef"=w245:refnum<vi>, "NewVal"=w243:string)  [unwired: 1 in]
        n138 = call <vilib>:"WPI_UtilitiesGetTreeIOName.vi"("NewVal"=w243, "TreeControl in"=w245) -> ("I/O Name"=w246:string)  [unwired: 9 in]
        n139 = case shown="\"Analog Out\", \"Motor\", \"PWM\"" w246 {
          selector: w246 -> [_ w253 _ w275 w284 _]
          tunnel: w243 -> [_ _ w272 w274 _ w291]
          tunnel: w242 -> [_ _ _ _ _ w290]
          frame Default {
            w248 = FALSE ("Visible")
            w247 = FALSE ("Visible")
            n140 = property on="Motor" class="Clust (strict)"("Visible"=w247) -> ()  [unwired: 2 in, 2 out]
            n141 = property on="Test Ring" class="Ring (strict)"("Visible"=w247) -> ()  [unwired: 2 in, 2 out]
            n142 = property on="Rev/Fwd" class="Clust (strict)"("Visible"=w248) -> ()  [unwired: 2 in, 2 out]
            n143 = property on="On/Off" class="Bool (strict)"("Visible"=w248) -> ()  [unwired: 2 in, 2 out]
            n144 = property on="Test Slider" class="Slide (strict)"("Visible"=w248) -> ()  [unwired: 2 in, 2 out]
          }
          frame "Analog Out", "Motor", "PWM" {
            w254 = FALSE ("Visible")
            n145 = case shown="\"Analog Out\"" w253 {
              tunnel: [1.0 ("Value") -1.0 ("Value") 0.0 ("Value")] -> w252
              tunnel: [255.0 ("Value") 1.0 ("Value") 5.0 ("Value")] -> w251
              tunnel: [128.0 ("Value") 0.0 ("Value") 0.0 ("Value")] -> w250
              tunnel: [64.0 ("Value") 0.5 ("Value") 1.0 ("Value")] -> w249
              frame "PWM" {
              }
              frame "Motor", Default {
              }
              frame "Analog Out" {
              }
            }
            n146 = property on="Motor" class="Clust (strict)"("Visible"=TRUE) -> ()  [unwired: 2 in, 2 out]
            n147 = property on="Value" class="Slide (strict)"("Value"=w250, "Scale.Minimum"=w252, "Scale.Maximum"=w251, "Scale.Increment"=w249) -> ()  [unwired: 2 in, 2 out]
            n148 = property on="On/Off" class="Bool (strict)"("Visible"=w254) -> ()  [unwired: 2 in, 2 out]
            n149 = property on="Test Slider" class="Slide (strict)"("Visible"=w254) -> ()  [unwired: 2 in, 2 out]
            n150 = property on="Test Ring" class="Ring (strict)"("Visible"=w254) -> ()  [unwired: 2 in, 2 out]
            n151 = property on="Rev/Fwd" class="Clust (strict)"("Visible"=w254) -> ()  [unwired: 2 in, 2 out]
          }
          frame "Servo" {
            w270 = FALSE ("Visible")
            n152 = call <vilib>:"NT Read Number.vi"("Name"=w272) -> ("Numeric"=w271:dbl)  [unwired: 9 in, 1 out]
            n153 = property on="Test Slider" class="Slide (strict)"("Visible"=TRUE, "Scale.Maximum"=170.0 ("Scale.Range:Maximum")) -> ()  [unwired: 2 in, 2 out]
            n154 = local write "Test Slider"(w271) -> ()
            n155 = property on="Motor" class="Clust (strict)"("Visible"=w270) -> ()  [unwired: 2 in, 2 out]
            n156 = property on="Rev/Fwd" class="Clust (strict)"("Visible"=w270) -> ()  [unwired: 2 in, 2 out]
            n157 = property on="On/Off" class="Bool (strict)"("Visible"=w270) -> ()  [unwired: 2 in, 2 out]
            n158 = property on="Test Ring" class="Ring (strict)"("Visible"=w270) -> ()  [unwired: 2 in, 2 out]
          }
          frame "Relay", "Solenoid" {
            w273 = FALSE ("Visible")
            n159 = property on="Motor" class="Clust (strict)"("Visible"=w273) -> ()  [unwired: 2 in, 2 out]
            n160 = property on="Test Slider" class="Slide (strict)"("Visible"=w273) -> ()  [unwired: 2 in, 2 out]
            n161 = Search and Replace String(input string=w274, search string="/Value  **", replace string="/Direction") -> (result string=w280:string)  [unwired: 5 in, 3 out]
            n162 = property on="Test Ring" class="Ring (strict)"("Visible"=w273) -> ()  [unwired: 2 in, 2 out]
            n163 = call <vilib>:"NT Read String.vi"("Name"=w280) -> ("String"=w278:string)  [unwired: 9 in, 1 out]
            n164 = Equal?(x="Both directions", y=w278) -> (x = y?=w276:bool)
            n165 = Not(x=w276) -> (.not. x?=w277:bool)
            n166 = property on="Rev/Fwd" class="Clust (strict)"("Visible"=w276) -> ()  [unwired: 2 in, 2 out]
            n167 = property on="On/Off" class="Bool (strict)"("Visible"=w277, "Caption.Text"=w275) -> ()  [unwired: 2 in, 2 out]
          }
          frame "Compressor", "Digital Out" {
            w283 = FALSE ("Visible")
            # "Get direction and finish"
            n168 = property on="Motor" class="Clust (strict)"("Visible"=w283) -> ()  [unwired: 2 in, 2 out]
            n169 = property on="Test Slider" class="Slide (strict)"("Visible"=w283) -> ()  [unwired: 2 in, 2 out]
            n170 = property on="Test Ring" class="Ring (strict)"("Visible"=w283) -> ()  [unwired: 2 in, 2 out]
            n171 = property on="On/Off" class="Bool (strict)"("Visible"=TRUE, "Caption.Text"=w284) -> ()  [unwired: 2 in, 2 out]
            n172 = property on="Rev/Fwd" class="Clust (strict)"("Visible"=FALSE) -> ()  [unwired: 2 in, 2 out]
          }
          frame "Camera" {
            n173 = call <vilib>:"Get Last Path Segment.vi"("String in"=w291) -> ("String out"=w292:string)  [unwired: 10 in]
            n174 = property on="On/Off" class="Bool (strict)"("Visible"=FALSE) -> ()  [unwired: 2 in, 2 out]
            n175 = property on="Motor" class="Clust (strict)"("Visible"=FALSE) -> ()  [unwired: 2 in, 2 out]
            n176 = property on="Rev/Fwd" class="Clust (strict)"("Visible"=FALSE) -> ()  [unwired: 2 in, 2 out]
            n177 = case shown="\"White Balance  **\"" w292 {
              tunnel: w291 -> [w298 w307 w316 w325 w334 _ w340]
              tunnel: w290 -> [w296 w304 w313 w322 w331 _ _]
              frame "Size  **" {
                n178 = Index Array(array=w296) -> (element=w295:cluster{string[]})  [unwired: 1 in]
                n179 = call <vilib>:"NT Read String.vi"("Name"=w298) -> ("String"=w297:string)  [unwired: 9 in, 1 out]
                n180 = Unbundle(w295) -> (w293:string[])
                n181 = Match First String(2:w293, 3:w297) -> (0:w294:i32)  [unwired: 1 out]
                n182 = property on="Test Ring" class="Ring (strict)"("Value"=w294, "Strings []"=w293) -> ()  [unwired: 2 in, 2 out]
                n183 = property on="Test Ring" class="Ring (strict)"("Visible"=TRUE) -> ()  [unwired: 2 in, 2 out]
                n184 = property on="Test Slider" class="Slide (strict)"("Visible"=FALSE) -> ()  [unwired: 2 in, 2 out]
              }
              frame "White Balance  **" {
                n185 = Index Array(array=w304, index=1) -> (element=w305:cluster{string[]})
                n186 = call <vilib>:"NT Read String.vi"("Name"=w307) -> ("String"=w306:string)  [unwired: 9 in, 1 out]
                n187 = Unbundle(w305) -> (w302:string[])
                n188 = Match First String(2:w302, 3:w306) -> (0:w301:i32)  [unwired: 1 out]
                n189 = property on="Test Ring" class="Ring (strict)"("Value"=w301, "Strings []"=w302) -> ()  [unwired: 2 in, 2 out]
                n190 = property on="Test Ring" class="Ring (strict)"("Visible"=TRUE) -> ()  [unwired: 2 in, 2 out]
                n191 = property on="Test Slider" class="Slide (strict)"("Visible"=FALSE) -> ()  [unwired: 2 in, 2 out]
              }
              frame "Exposure  **" {
                n192 = Index Array(array=w313, index=2) -> (element=w314:cluster{string[]})
                n193 = call <vilib>:"NT Read String.vi"("Name"=w316) -> ("String"=w315:string)  [unwired: 9 in, 1 out]
                n194 = Unbundle(w314) -> (w310:string[])
                n195 = Match First String(2:w310, 3:w315) -> (0:w311:i32)  [unwired: 1 out]
                n196 = property on="Test Ring" class="Ring (strict)"("Value"=w311, "Strings []"=w310) -> ()  [unwired: 2 in, 2 out]
                n197 = property on="Test Ring" class="Ring (strict)"("Visible"=TRUE) -> ()  [unwired: 2 in, 2 out]
                n198 = property on="Test Slider" class="Slide (strict)"("Visible"=FALSE) -> ()  [unwired: 2 in, 2 out]
              }
              frame "Exposure Priority  **" {
                n199 = Index Array(array=w322, index=3) -> (element=w323:cluster{string[]})
                n200 = call <vilib>:"NT Read String.vi"("Name"=w325) -> ("String"=w324:string)  [unwired: 9 in, 1 out]
                n201 = Unbundle(w323) -> (w319:string[])
                n202 = Match First String(2:w319, 3:w324) -> (0:w320:i32)  [unwired: 1 out]
                n203 = property on="Test Ring" class="Ring (strict)"("Value"=w320, "Strings []"=w319) -> ()  [unwired: 2 in, 2 out]
                n204 = property on="Test Ring" class="Ring (strict)"("Visible"=TRUE) -> ()  [unwired: 2 in, 2 out]
                n205 = property on="Test Slider" class="Slide (strict)"("Visible"=FALSE) -> ()  [unwired: 2 in, 2 out]
              }
              frame "Color Enable  **" {
                n206 = Index Array(array=w331, index=4) -> (element=w332:cluster{string[]})
                n207 = call <vilib>:"NT Read String.vi"("Name"=w334) -> ("String"=w333:string)  [unwired: 9 in, 1 out]
                n208 = Unbundle(w332) -> (w328:string[])
                n209 = Match First String(2:w328, 3:w333) -> (0:w329:i32)  [unwired: 1 out]
                n210 = property on="Test Ring" class="Ring (strict)"("Value"=w329, "Strings []"=w328) -> ()  [unwired: 2 in, 2 out]
                n211 = property on="Test Ring" class="Ring (strict)"("Visible"=TRUE) -> ()  [unwired: 2 in, 2 out]
                n212 = property on="Test Slider" class="Slide (strict)"("Visible"=FALSE) -> ()  [unwired: 2 in, 2 out]
              }
              frame Default {
                n213 = property on="Test Ring" class="Ring (strict)"("Visible"=FALSE) -> ()  [unwired: 2 in, 2 out]
                n214 = property on="Test Slider" class="Slide (strict)"("Visible"=FALSE) -> ()  [unwired: 2 in, 2 out]
              }
              frame "Brightness  **", "Color Level  **", "Compression  **", "FPS  **", "Sharpness  **" {
                n215 = call <vilib>:"NT Read Number.vi"("Name"=w340) -> ("Numeric"=w339:dbl)  [unwired: 9 in, 1 out]
                n216 = local write "Test Slider"(w339) -> ()
                n217 = property on="Test Slider" class="Slide (strict)"("Visible"=TRUE, "Scale.Maximum"=100.0 ("Scale.Range:Maximum")) -> ()  [unwired: 2 in, 2 out]
                n218 = property on="Test Ring" class="Ring (strict)"("Visible"=FALSE) -> ()  [unwired: 2 in, 2 out]
              }
            }
          }
        }
        n219 = property on="Progress" class="Clust (strict)"("Visible"=FALSE) -> ()  [unwired: 2 in, 2 out]
      }
      event "Test Name": Mouse Enter {
        # "Populate the ring with the list of tests"
        n220 = event-data() -> ()  [unwired: 1 in, 1 out]
        n221 = call <vilib>:"NT Read String Array.vi"("Name"="/TestMode/TestList") -> ("String Array"=w349:string[])  [unwired: 9 in, 1 out]
        n222 = Build Array (concatenate)("Select the test to run...", w349) -> (w348:string[])
        n223 = property on="Test Name" class="Ring (strict)"("Strings []"=w348) -> ()  [unwired: 2 in, 2 out]
      }
      event "Test Name": Value Change {
        w352 = FALSE ("Visible")
        # "Tell the robot the test name to run"
        n224 = event-data() -> ("NewVal"=w356:u16)  [unwired: 1 in]
        n225 = property on="Test Name" class="Ring (strict)"() -> ("Strings []"=w357:string[])  [unwired: 2 in, 2 out]
        n226 = local write "Progress"(T6 {"Test Progress"=0, "Test Progress Text"=""} ("Progress")) -> ()
        n227 = Index Array(array=w357, index=w356) -> (element=w355:string)
        n228 = call <vilib>:"NT Write String.vi"("String"=w355, "Name"="/TestMode/TestName") -> ()  [unwired: 9 in, 1 out]
        n229 = property on="Progress" class="Clust (strict)"("Visible"=TRUE) -> ()  [unwired: 2 in, 2 out]
        n230 = property on="Motor" class="Clust (strict)"("Visible"=w352) -> ()  [unwired: 2 in, 2 out]
        n231 = property on="Test Slider" class="Slide (strict)"("Visible"=w352) -> ()  [unwired: 2 in, 2 out]
        n232 = property on="On/Off" class="Bool (strict)"("Visible"=w352) -> ()  [unwired: 2 in, 2 out]
        n233 = property on="Rev/Fwd" class="Clust (strict)"("Visible"=w352) -> ()  [unwired: 2 in, 2 out]
        n234 = property on="Test Ring" class="Ring (strict)"("Visible"=w352) -> ()  [unwired: 2 in, 2 out]
      }
      event "Select Auto": Mouse Enter {
        # "Populate the combo box with the list of autonomous options"
        n235 = event-data() -> ()  [unwired: 1 in, 1 out]
        n236 = call <vilib>:"NT Read String Array.vi"("Name"="Auto List") -> ("String Array"=w359:string[])  [unwired: 9 in, 1 out]
        n237 = property on="Select Auto" class="CmbBox"("Strings[]"=w359) -> ()  [unwired: 2 in, 2 out]
      }
      event "Select Auto": Value Change {
        # "User modified the Auto Selection. Write to NT variable so robot knows."
        n238 = event-data() -> ("NewVal"=w363:string)  [unwired: 1 in]
        n239 = call <vilib>:"NT Write String.vi"("String"=w363, "Name"="Auto Selector") -> ()  [unwired: 9 in, 1 out]
      }
      event "Command Selection": Value Change {
        # "Get the params and show in table"
        n240 = event-data() -> ("NewVal"=w370:i32)  [unwired: 1 in]
        n241 = property on="Command Selection" class="MCListbox (strict)"() -> ("ItemNames"=w368:string[][])  [unwired: 2 in, 2 out]
        n242 = call <vilib>:"WPI_DashboardUpdate Command Params.vi"("NewVal"=w370, "Commands"=w368, "Param Tbl"=w369) -> ()  [unwired: 8 in, 1 out]
      }
      event "Execute Command": Value Change {
        # "Started one, Unique ID holds\nresponse"
        n243 = event-data() -> ()  [unwired: 1 in, 1 out]
        n244 = property on="Command Selection" class="MCListbox (strict)"() -> ("ItemNames"=w382:string[][])  [unwired: 2 in, 2 out]
        n245 = Index Array(array=w382, index (row)="Command Selection", index (col)=0) -> (element=w380:string)
        n246 = call <vilib>:"Invoke Commands.vi"("Command Params"="Command Params", "Function Name"=w380) -> ("Params"=w376:u8, "Started"=w375:bool)  [unwired: 7 in, 1 out]
        n247 = Array Subset(array="Command Params", length (row)=w376) -> (w377:string[][])  [unwired: 3 in]
        n248 = Select(t="Executing" ("Cmd Status"), s=w375, f="" ("Cmd Status")) -> (s? t:f=→"Cmd Status":string)
      }
      event "Command Selection": Double Click {
        n249 = event-data() -> ("Row"=w392:i32)  [unwired: 1 in]
        n250 = property on="Command Selection" class="MCListbox (strict)"() -> ("ItemNames"=w395:string[][])  [unwired: 2 in, 2 out]
        n251 = local read "Command Params"() -> (w390:string[][])
        n252 = Index Array(array=w395, index (row)=w392, index (col)=0) -> (element=w393:string)
        n253 = call <vilib>:"Invoke Commands.vi"("Command Params"=w390, "Function Name"=w393) -> ("Params"=w389:u8, "Started"=w384:bool)  [unwired: 7 in, 1 out]
        n254 = Array Subset(array=w390, length (row)=w389) -> (w388:string[][])  [unwired: 3 in]
        n255 = Select(t="Executing" ("Cmd Status"), s=w384, f="" ("Cmd Status")) -> (s? t:f=w385:string)
        n256 = local write "Cmd Status"(w385) -> ()
      }
      event "CheckList": Double Click {
        # "Shift clears all"
        # "Update symbols on the listbox"
        n257 = event-data() -> ("PlatMods.Shift"=w398:bool, "Row"=w400:i32)  [unwired: 1 in]
        n258 = case shown="True" w398 {
          tunnel: w400 -> [w404 _]
          tunnel: 1 -> [w403 _]
          frame False {
            n259 = property on="CheckList" class="LstBox (strict)"() -> ("Item Symbols"=w402:i32[])  [unwired: 2 in, 2 out]
            n260 = Replace Array Subset(array=w402, new element=w403, index=w404) -> (w401:i32[])
            n261 = property on="CheckList" class="LstBox (strict)"("Item Symbols"=w401) -> ()  [unwired: 2 in, 2 out]
          }
          frame True {
            w405 = 0 ("Top Row")
            n262 = property on="CheckList" class="LstBox (strict)"() -> ("Number of Rows"=w407:u32)  [unwired: 2 in, 2 out]
            n263 = Initialize Array(0, w407) -> (w406:i32[])
            n264 = property on="CheckList" class="LstBox (strict)"("Top Row"=w405, "Value"=w405, "Item Symbols"=w406) -> ()  [unwired: 2 in, 2 out]
          }
        }
      }
      event "CheckList": Key Down {
        # "Update symbols on the listbox\nLeft and right keys check and uncheck"
        n265 = event-data() -> ("VKey"=w412:T18)  [unwired: 1 in]
        n266 = case shown="\"Left\", \"Right\"" w412 {
          selector: w412 -> [w417 _]
          tunnel: eventvkey."Left" ("VKey") -> [w415 _]
          frame "Left", "Right" {
            n267 = Equal?(x=w415, y=w417) -> (x = y?=w416:bool)
            n268 = Select(t=0, s=w416, f=1) -> (s? t:f=w418:i32)
            n269 = property on="CheckList" class="LstBox (strict)"() -> ("Item Symbols"=w421:i32[])  [unwired: 2 in, 2 out]
            n270 = Replace Array Subset(array=w421, new element=w418, index="CheckList") -> (w420:i32[])
            n271 = property on="CheckList" class="LstBox (strict)"("Item Symbols"=w420) -> ()  [unwired: 2 in, 2 out]
          }
          frame Default {
          }
        }
      }
      event "DB Camera Config": Value Change {
        # "Show or hide the cluster of controls, store in ini file"
        n272 = event-data() -> ("NewVal"=w426:bool)  [unwired: 1 in]
        n273 = case shown="False" w426 {
          tunnel: w425 -> [w435 _]
          tunnel: [w428 w446] -> w424
          tunnel: w423 -> [w427 w446]
          frame False {
            w442 = "Camera"
            w445 = FALSE ("Visible")
            n274 = local read "Camera Settings"() -> (w434:T4)
            n275 = Index Array(array=w435) -> (element=w438:cluster{string[]})  [unwired: 1 in]
            n276 = Unbundle(w434) -> ("Frame Rate"=w433:i32, "Compression"=w432:i32, "Size"=w436:u16)
            n277 = Unbundle(w438) -> (w437:string[])
            n278 = Index Array(array=w437, index=w436) -> (element=w431:string)
            n279 = call-poly <vilib>:"Write Key.vi"("section"=w442, "value"=w431, "key"="Size", "refnum"=w427) -> ("refnum out"=w444:T12)  [unwired: 2 in, 5 out]
            n280 = call-poly <vilib>:"Write Key.vi"("section"=w442, "value"=w433, "key"="FrameRate", "refnum"=w444) -> ("refnum out"=w443:T12)  [unwired: 1 in, 6 out]
            n281 = property on="Camera Settings" class="Clust (strict)"("Visible"=w445) -> ()  [unwired: 2 in, 2 out]
            n282 = local write "DB Camera Config"(w445) -> ()
            n283 = call-poly <vilib>:"Write Key.vi"("section"=w442, "value"=w432, "key"="Compression", "refnum"=w443) -> ("refnum out"=w429:T12)  [unwired: 1 in, 6 out]
            n284 = call <vilib>:"Close Config Data.vi"("refnum"=w429) -> ("file path"=w430:path)  [unwired: 2 in, 8 out]
            n285 = call <vilib>:"Open Config Data.vi"("configuration file path"=w430) -> ("refnum"=w428:T12)  [unwired: 8 in, 2 out]
          }
          frame True {
            n286 = property on="Camera Settings" class="Clust (strict)"("Visible"=TRUE) -> ()  [unwired: 2 in, 2 out]
          }
        }
      }
      event "Camera Settings": Value Change {
        # "Update summary string when any elements of DB camera change"
        n287 = event-data() -> ("NewVal"=w460:T4)  [unwired: 1 in]
        n288 = Index Array(array=w456) -> (element=w455:cluster{string[]})  [unwired: 1 in]
        n289 = Unbundle(w460) -> ("Frame Rate"=w451:i32, "Compression"=w450:i32, "Size"=w453:u16)
        n290 = Unbundle(w455) -> (w454:string[])
        n291 = Index Array(array=w454, index=w453) -> (element=w452:string)
        n292 = Format Into String(format string="%s   %dfps   %d%%", w452, w451, w450) -> (resulting string=w457:string)  [unwired: 2 in, 1 out]
        n293 = Build Array(w457) -> (w458:string[])
        n294 = property on="DB Camera Config" class="Bool (strict)"("Strings [4]"=w458) -> ()  [unwired: 2 in, 2 out]
      }
      event "Motor.Enable": Value Change {
        # "When the test mode otor enable helper is set, update that\ntree row item's value"
        n295 = event-data() -> ("NewVal"=w467:bool)  [unwired: 1 in]
        n296 = Unbundle("Motor") -> ("Value"=w466:dbl)  [unwired: 1 out]
        n297 = Select(t=w466, s=w467, f=0.0) -> (s? t:f=w464:dbl)
        n298 = call <vilib>:"NT Write Number.vi"("Numeric"=w464, "Name"=w463) -> ()  [unwired: 9 in, 1 out]
      }
      event "Test Slider": Value Change {
        # "When the test mode slider helper is set, update that\ntree row item's value"
        n299 = event-data() -> ("NewVal"=w471:dbl)  [unwired: 1 in]
        n300 = call <vilib>:"NT Write Number.vi"("Numeric"=w471, "Name"=w472) -> ()  [unwired: 9 in, 1 out]
      }
      event "On/Off": Value Change {
        # "When the test mode on/off helper value is set, update that\ntree row item's value"
        n301 = event-data() -> ("NewVal"=w477:bool)  [unwired: 1 in]
        n302 = Boolean To (0,1)(Boolean=w477) -> (0, 1=w476:i16)
        n303 = call <vilib>:"NT Write Number.vi"("Numeric"=w476, "Name"=w475) -> ()  [unwired: 9 in, 1 out]
      }
      event "Rev/Fwd": Value Change {
        # "When the test mode helper value for relays is set, update that\ntree row item's value"
        n304 = event-data() -> ("NewVal.Forward"=w486:bool, "NewVal.Reverse"=w485:bool)  [unwired: 1 in]
        n305 = Boolean To (0,1)(Boolean=w486) -> (0, 1=w482:i16)
        n306 = Boolean To (0,1)(Boolean=w485) -> (0, 1=w484:i16)
        n307 = Negate(x=w484) -> (-x=w483:i16)
        n308 = Add(x=w482, y=w483) -> (x+y=w481:i16)
        n309 = call <vilib>:"NT Write Number.vi"("Numeric"=w481, "Name"=w480) -> ()  [unwired: 9 in, 1 out]
      }
      event "Test Ring": Value Change {
        # "When a test mode helper value is selected from the ring,\nset the tree item's variable to the string value"
        n310 = event-data() -> ("NewVal"=w491:u16)  [unwired: 1 in]
        n311 = property on="Test Ring" class="Ring (strict)"() -> ("Strings []"=w492:string[])  [unwired: 2 in, 2 out]
        n312 = Index Array(array=w492, index=w491) -> (element=w490:string)
        n313 = call <vilib>:"NT Write String.vi"("String"=w490, "Name"=w489) -> ()  [unwired: 9 in, 1 out]
      }
      event "Rec Mode": Value Change {
        # "Update globals for recording mode and path to read log from.\nClear when logging and let NetworkTables set path for vision to\nuse."
        n314 = event-data() -> ("NewVal"=w502:enum32{"Stop", "Record", "Playback"})  [unwired: 1 in]
        n315 = global write "WPI_DashboardLogging Global.vi" "Logging Filename"(path "") -> ()
        n316 = global write "WPI_DashboardLogging Global.vi" "Recording"(w502) -> ()
        n317 = case shown="\"Playback\"" w502 {
          tunnel: w501 -> [_ w504 w513]
          tunnel: [_ _ w512] -> w498
          tunnel: [_ _ w511] -> _
          tunnel: w496 -> [_ _ w509]
          tunnel: cluster{i32, i32} {-250, 170} -> [_ _ w508]
          tunnel: [_ _ T19 {"Image Size"=TRUE, "Image Type"=TRUE, "Pixel Value"=TRUE, "ROI Information"=TRUE, "Zoom Factor"=FALSE} ("Image Information Shown:All Elements")] -> _
          tunnel: [_ _ TRUE ("Zoom Factor")] -> _
          tunnel: w494 -> [_ _ w505]
          frame Default {
          }
          frame "Stop", "Record" {
            # "Place Window too"
            n318 = invoke class="VI" method="FP.Close"(reference=w504) -> (reference out=w503:refnum<vi>)  [unwired: 2 in, 2 out]
            n319 = invoke class="VI" method="Abort VI"(reference=w503) -> ()  [unwired: 2 in, 3 out]
          }
          frame "Playback" {
            n320 = call "Open Playback Panel.vi"("Offset"=w508, "DB VI Ref"=w509, "Playback in"=w513) -> ("Playback out"=w510:refnum<vi>)  [unwired: 8 in]
            n321 = register-events(w510, w505) -> (reference out=w512:refnum<event-registration>, error out=w511:errorcluster)  [unwired: 2 in]
          }
        }
        n322 = call <vilib>:"WPI_DashboardNT Log FieldName Cache.vi"("Operation"=enum16{"Lookup/Add", "Index", "Clear"}."Clear") -> ()  [unwired: 8 in, 3 out]
      }
      event Panel Close {
        w515 = enum32{"Stop", "Record", "Playback"}."Stop" ("Rec Mode")
        # "Playback window has been closed, abort"
        n323 = event-data() -> ()  [unwired: 1 in, 4 out]
        n324 = local write "Rec Mode"(w515) -> ()
        n325 = global write "WPI_DashboardLogging Global.vi" "Recording"(w515) -> ()
      }
      event Panel Close {
        # "Abort playback window and ourself"
        n326 = event-data() -> ()  [unwired: 1 in, 4 out]
        n327 = invoke class="VI" method="FP.Close"(reference=w521) -> (reference out=w520:refnum<vi>)  [unwired: 2 in, 2 out]
        n328 = invoke class="VI" method="Abort VI"(reference=w520) -> (error out=w519:errorcluster)  [unwired: 2 in, 2 out]
        n329 = invoke class="VI" method="Abort VI"(error in=w519) -> ()  [unwired: 2 in, 3 out]
      }
      event User Event {
        n330 = event-data() -> ("IDs"=w529:cluster{"RPC field ID":u16, "Unique ID":u16}, "String"=w528:string)  [unwired: 1 in]
        n331 = Bundle("IDs"=w529, "String"=w528) -> (w527:T7)  [unwired: 1 in]
        n332 = call <vilib>:"Retrieve RPC Response.vi"("RPC Response"=w527) -> ("Output"=w524:string[][])  [unwired: 10 in]
        n333 = Build Array (concatenate)(w522, w524) -> (w523:string[][])
        n334 = local write "Command Params"(w523) -> ()
        n335 = local write "Cmd Status"("" ("Cmd Status")) -> ()
      }
      event "Vision": Value Change {
        # "Enable/Disable Compression slider.\nHW USB is hard-coded into the camera"
        n336 = event-data() -> ("NewVal"=w536:u16)  [unwired: 1 in]
        n337 = Equal?(x=w536, y=u32 2 ("milliseconds to wait")) -> (x = y?=w534:bool)
        n338 = Select(t=T20."Disabled and Grayed Out" ("Disabled"), s=w534, f=T20."Enabled" ("Disabled")) -> (s? t:f=w531:T20)
        n339 = property on="Compression" class="Slide (strict)"("DisabledEnum"=w531) -> ()  [unwired: 2 in, 2 out]
      }
      event "Tree": Double Click {
        n340 = event-data() -> ("PlatMods"=w541:T23, "Tag"=w540:string)  [unwired: 1 in]
        n341 = Unbundle(w541) -> ("Shift"=w539:bool)  [unwired: 4 out]
        n342 = Not(x=w539) -> (.not. x?=w538:bool)
        n343 = call <vilib>:"NT Update Persistence.vi"("Persistence"=w538, "Name"=w540) -> ()  [unwired: 9 in, 1 out]
      }
    }
  }
  n344 = while {
    tunnel: w47 -> [w545]
    i -> [w548]
    stop <- FALSE stop-if-true
    n345 = Wait (ms)(milliseconds to wait=u32 100) -> ()  [unwired: 1 out]
    n346 = case shown="\"Playback\"" "Rec Mode" {
      tunnel: w548 -> [_ _ w563]
      tunnel: [u32 2829099 ("Base Color") u32 11141120 ("Target Color") w552] -> w544
      frame "Stop", Default {
        # "Reset the color, extra updates don't cost much"
      }
      frame "Record" {
      }
      frame "Playback" {
        # "Playback"
        n347 = Quotient & Remainder(x=w563, y=u32 50 ("milliseconds to wait")) -> (x-y*floor(x/y)=w559:u32)  [unwired: 1 out]
        n348 = Divide(x=w559, y=u32 50 ("milliseconds to wait")) -> (x/y=w556:dbl)
        n349 = Multiply(x=6.283185307179586, y=w556) -> (x*y=w561:dbl)
        n350 = Sine(x=w561) -> (sin(x)=w560:dbl)
        n351 = Absolute Value(x=w560) -> (abs(x)=w553:dbl)
        n352 = call "Interpolate RGB Color.vi"("Proportion"=w553, "Target Color"=u32 30976, "Base Color"=u32 2829099) -> ("Result Color"=w552:u32)  [unwired: 8 in]
      }
    }
    n353 = property class="Pane"(reference=w545, "PaneColor"=w544) -> ()  [unwired: 1 in, 2 out]
  }
  n354 = property on="On/Off" class="Bool (strict)"("Visible"=w19) -> ()  [unwired: 2 in, 2 out]
  n355 = property on="Motor" class="Clust (strict)"("Visible"=w19) -> ()  [unwired: 2 in, 2 out]
  n356 = property on="Progress" class="Clust (strict)"("Visible"=w19) -> ()  [unwired: 2 in, 2 out]
  n357 = property on="Test Ring" class="Ring (strict)"("Visible"=w19) -> ()  [unwired: 2 in, 2 out]
  n358 = property on="Rev/Fwd" class="Clust (strict)"("Visible"=w19) -> ()  [unwired: 2 in, 2 out]
  n359 = property on="Camera Settings" class="Clust (strict)"("Visible"=w19) -> ()  [unwired: 2 in, 2 out]
  n360 = local write "DB Camera Config"(w19) -> ()
  n361 = local write "Command Params"(string[][] [] ("Command Params")) -> ()
  n362 = global write "WPI_DashboardLogging Global.vi" "Recording"(w41) -> ()
  n363 = local write "Rec Mode"(w41) -> ()
  n364 = while {
    tunnel: u16 1741 ("timeout ms (25000)") -> [w565]
    stop <- FALSE stop-if-true
    n365 = TCP Create Listener(10:w565) -> (0:w564:errorcluster, 3:w566:refnum<k5>)  [unwired: 4 in, 1 out]
    n366 = case shown="No Error" w564 {
      selector: w564 -> [w568 _]
      tunnel: w566 -> [w569 _]
      frame No Error {
        n367 = while {
          tunnel: w569 -> [w572]
          tunnel: w568 -> [w571]
          stop <- FALSE stop-if-true
          n368 = TCP Wait On Listener(8:w571, 11:w572) -> (0:w573:errorcluster, 4:w574:refnum<k5>)  [unwired: 2 in, 3 out]
          n369 = local write "TCP"(w574) -> ()
          n370 = case shown="No Error" w573 {
            frame No Error {
            }
            frame Error {
              n371 = Wait (ms)(milliseconds to wait=u32 1000) -> ()  [unwired: 1 out]
            }
          }
        }
      }
      frame Error {
        n372 = Wait (ms)(milliseconds to wait=u32 1000) -> ()  [unwired: 1 out]
      }
    }
  }
  n373 = local write "Command Selection"(u16 0 ("milliseconds to wait")) -> ()
